vi "SLSC Read Properties.vi"(0 "session in":refnum<k21>, 1 "LoopDuration(ms)":dbl, 5 "SLSC Module Name":refnum<k21>, 11 "error in":errorcluster, 12 "SLSC Dynamic Inputs":T1[](array[typedef])) -> (4 "session out":refnum<k21>, 6 "SLSC Module Name":refnum<k21>, 8 "Values":dbl[](array[numeric]), 15 "error out":errorcluster)   [LabVIEW 2015, in "SLSC CD Engine.lvlib"]
uses:
  SLSC CD Engine.lvlib
  SLSC Dynamic Channel.ctl
  SLSC Datatype.ctl
  <vilib>/SLSC/Get Generic Property (U64).vi
  <vilib>/SLSC/Get Generic Property (U32).vi
  <vilib>/SLSC/Get Generic Property (String).vi
  <vilib>/SLSC/Get Generic Property (I64).vi
  <vilib>/SLSC/Get Generic Property (I32).vi
  <vilib>/SLSC/Get Generic Property (DBL).vi
  <vilib>/SLSC/Get Generic Property (Bool).vi
  <vilib>/SLSC/SLSC.lvlib
  SLSC CD Shared/SLSC CD Shared.lvlib
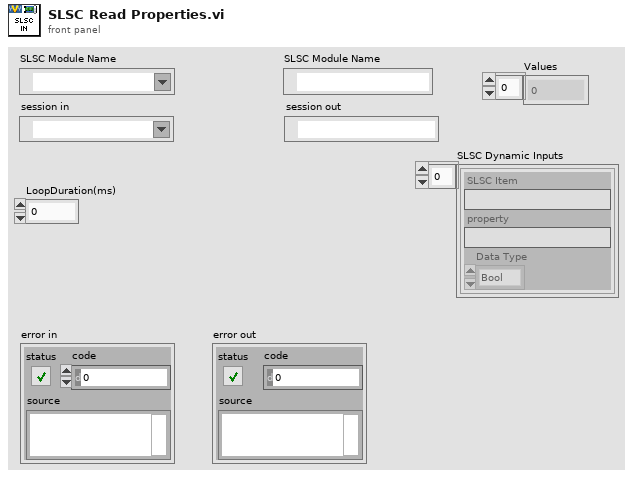
[diagram p1: front panel]
types:
  T1 = typedef "SLSC CD Shared.lvlib/SLSC Dynamic Channel.ctl" = cluster{"SLSC Item":string, "property":string, "Data Type":T2}
  T2 = typedef "SLSC CD Shared.lvlib/SLSC Datatype.ctl" = enum16{"Bool", "Double", "I32", "I64", "String", "U32", "U64"}
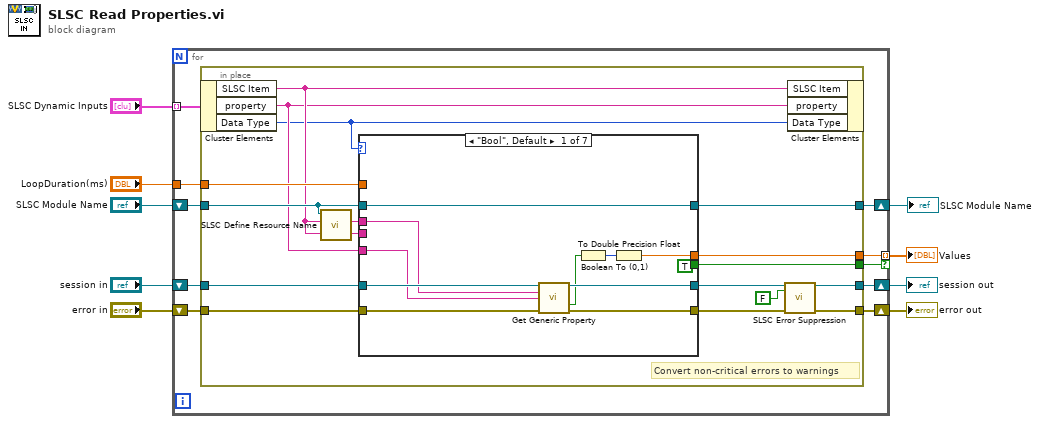
[diagram p0: block diagram]
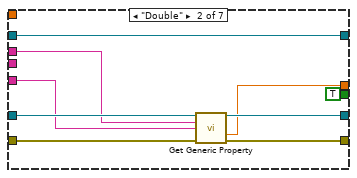
[diagram p2: hidden frame]
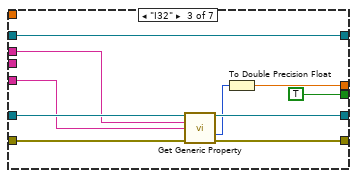
[diagram p3: hidden frame]
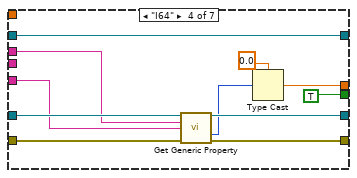
[diagram p4: hidden frame]
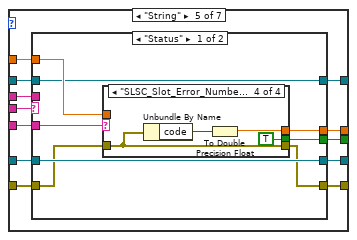
[diagram p5: hidden frame]
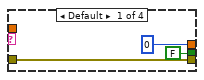
[diagram p6: hidden frame]
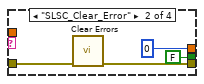
[diagram p7: hidden frame]
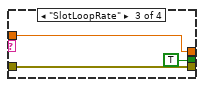
[diagram p8: hidden frame]
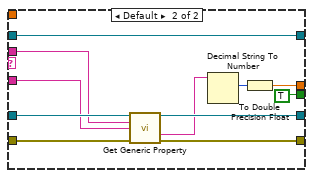
[diagram p9: hidden frame]
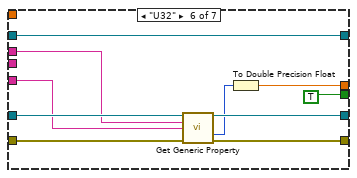
[diagram p10: hidden frame]
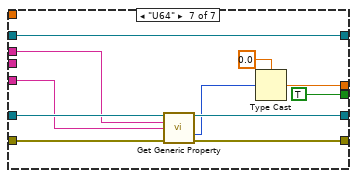
[diagram p11: hidden frame]
diagram:
  n1 = for {
    tunnel: "SLSC Dynamic Inputs" -> [w10] mode=indexing
    shift-right: [w16] -> w7
    shift-left: "session in" -> [w19]
    shift-right: [w14] -> w4
    shift-left: "SLSC Module Name" -> [w11]
    tunnel: [w17] -> w3 mode=indexing if=w13
    tunnel: "LoopDuration(ms)" -> [w12]
    shift-right: [w15] -> w9
    shift-left: "error in" -> [w18]
    n2 = in-place {
      in-place-border: w19 -> [w34]
      in-place-border: w18 -> [w33]
      in-place-border: [w32] -> w17
      in-place-border: [w31] -> w16
      in-place-border: [w20] -> w15
      in-place-border: [w30] -> w14
      in-place-border: [w29] -> w13
      in-place-border: w12 -> [w28]
      in-place-border: w11 -> [w27]
      # "Convert non-critical errors to warnings"
      n3 = in-place-cluster #1(w10) -> ("SLSC Item"=w25:string, "property"=w24:string, "Data Type"=w23:T2)
      n4 = call "SLSC Define Resource Name.vi"("SLSC Item"=w25, "SLSC Module Name"=w27) -> ("Resource"=w26:string)  [unwired: 9 in]
      n5 = case shown="\"Bool\", Default" w23 {
        tunnel: w34 -> [w45 w54 w64 w75 w87 w130 w141]
        tunnel: [w44 w53 w63 w74 w86 w129 w140] -> w31
        tunnel: w24 -> [w43 w52 w62 w73 w85 w128 w139]
        tunnel: w25 -> [_ _ _ _ w81 _ _]
        tunnel: w27 -> [w42 w51 w61 w72 w79 w127 w138]
        tunnel: [w42 w51 w61 w72 w77 w127 w138] -> w30
        tunnel: w33 -> [w41 w50 w60 w71 w84 w126 w137]
        tunnel: [w40 w49 w59 w70 w83 w125 w136] -> w21
        tunnel: [w37 w48 w58 w69 w82 w124 w135] -> w32
        tunnel: [TRUE TRUE TRUE TRUE w80 TRUE TRUE] -> w29
        tunnel: w28 -> [_ _ _ _ w78 _ _]
        tunnel: w26 -> [w35 w46 w55 w65 w76 w121 w131]
        frame "Bool", Default {
          n6 = call-poly <vilib>:"Get Generic Property.vi"("session in"=w45, "resources"=w35, "property"=w43, "error in (no error)"=w41) -> ("session out"=w44:refnum<k21>, "property value"=w39:bool, "error out"=w40:errorcluster)  [unwired: 9 in]
          n7 = Boolean To (0,1)(Boolean=w39) -> (0, 1=w38:i16)
          n8 = To Double Precision Float(number=w38) -> (double precision float=w37:dbl)
        }
        frame "Double" {
          n9 = call-poly <vilib>:"Get Generic Property.vi"("session in"=w54, "resources"=w46, "property"=w52, "error in (no error)"=w50) -> ("session out"=w53:refnum<k21>, "property value"=w48:dbl, "error out"=w49:errorcluster)  [unwired: 9 in]
        }
        frame "I32" {
          n10 = call-poly <vilib>:"Get Generic Property.vi"("session in"=w64, "resources"=w55, "property"=w62, "error in (no error)"=w60) -> ("session out"=w63:refnum<k21>, "property value"=w57:i32, "error out"=w59:errorcluster)  [unwired: 9 in]
          n11 = To Double Precision Float(number=w57) -> (double precision float=w58:dbl)
        }
        frame "I64" {
          n12 = call-poly <vilib>:"Get Generic Property.vi"("session in"=w75, "resources"=w65, "property"=w73, "error in (no error)"=w71) -> ("session out"=w74:refnum<k21>, "property value"=w68:i64, "error out"=w70:errorcluster)  [unwired: 9 in]
          n13 = Type Cast(type=0.0, x=w68) -> (*(type *) &x=w69:dbl)
        }
        frame "String" {
          n14 = case shown="\"Status\"" w81 {
            tunnel: w87 -> [w95 w120]
            tunnel: [w95 w119] -> w86
            tunnel: w85 -> [w91 w118]
            tunnel: w79 -> [w90 w111]
            tunnel: w84 -> [w89 w117]
            tunnel: [w88 w116] -> w83
            tunnel: [w94 w115] -> w82
            tunnel: [w92 TRUE] -> w80
            tunnel: w78 -> [w93 _]
            tunnel: [w90 w111] -> w77
            tunnel: w76 -> [_ w110]
            frame "Status" {
              n15 = case shown="\"SLSC_Slot_Error_Number\"" w91 {
                tunnel: [u32 0 ("LoopDuration(ms)") u32 0 ("LoopDuration(ms)") w104 w107] -> w94
                tunnel: w93 -> [_ _ w104 _]
                tunnel: [FALSE FALSE TRUE TRUE] -> w92
                tunnel: w89 -> [w96 w100 w103 w106]
                tunnel: [w96 w99 w103 w106] -> w88
                frame Default {
                }
                frame "SLSC_Clear_Error" {
                  n16 = call <vilib>:"Clear Errors.vi"("error in (no error)"=w100) -> ("error out"=w99:errorcluster)  [unwired: 5 in, 1 out]
                }
                frame "SlotLoopRate" {
                }
                frame "SLSC_Slot_Error_Number" {
                  n17 = Unbundle By Name(w106) -> ("code"=w108:i32)
                  n18 = To Double Precision Float(number=w108) -> (double precision float=w107:dbl)
                }
              }
            }
            frame Default {
              n19 = call-poly <vilib>:"Get Generic Property.vi"("session in"=w120, "resources"=w110, "property"=w118, "error in (no error)"=w117) -> ("session out"=w119:refnum<k21>, "property value"=w114:string, "error out"=w116:errorcluster)  [unwired: 9 in]
              n20 = Decimal String To Number(string=w114) -> (number=w113:i32)  [unwired: 2 in, 1 out]
              n21 = To Double Precision Float(number=w113) -> (double precision float=w115:dbl)
            }
          }
        }
        frame "U32" {
          n22 = call-poly <vilib>:"Get Generic Property.vi"("session in"=w130, "resources"=w121, "property"=w128, "error in (no error)"=w126) -> ("session out"=w129:refnum<k21>, "property value"=w123:u32, "error out"=w125:errorcluster)  [unwired: 9 in]
          n23 = To Double Precision Float(number=w123) -> (double precision float=w124:dbl)
        }
        frame "U64" {
          n24 = call-poly <vilib>:"Get Generic Property.vi"("session in"=w141, "resources"=w131, "property"=w139, "error in (no error)"=w137) -> ("session out"=w140:refnum<k21>, "property value"=w134:u64, "error out"=w136:errorcluster)  [unwired: 9 in]
          n25 = Type Cast(type=0.0, x=w134) -> (*(type *) &x=w135:dbl)
        }
      }
      n26 = call "SLSC Error Suppression.vi"("error in (no error)"=w21, "Popup Error?"=FALSE) -> ("error out"=w20:errorcluster)  [unwired: 7 in, 1 out]
      n27 = in-place-cluster #1("SLSC Item"=w25, "property"=w24, "Data Type"=w23) -> ()  [unwired: 1 out]
    }
  }
  "error out" <- w9
  "Values" <- w3
  "session out" <- w7
  "SLSC Module Name" <- w4
